vi "readdaq_tensions.vi"(10 "error in (no error)":errorcluster, 11 "Refnum in":refnum<k21>) -> (2 "viconsync":dbl, 3 "Tension Sensors Data":dbl[](array[numeric]), 5 "error out":errorcluster)   [LabVIEW 2017]
uses:
  <vilib>/DAQmx/read.llb/DAQmx Read (Analog 1D DBL NChan 1Samp).vi
  <vilib>/DAQmx/miscellaneous.llb/DAQmx Fill In Error Info.vi
  <vilib>/ptbypt/NI_PtbyPt.lvlib
panel:
  out "filtered":dbl[](array[numeric])
  out "Waveform Chart 2":dbl[](graph)
  in  "taresensors":bool
  out "raw data":dbl[](array[numeric]) format="%0.2f"
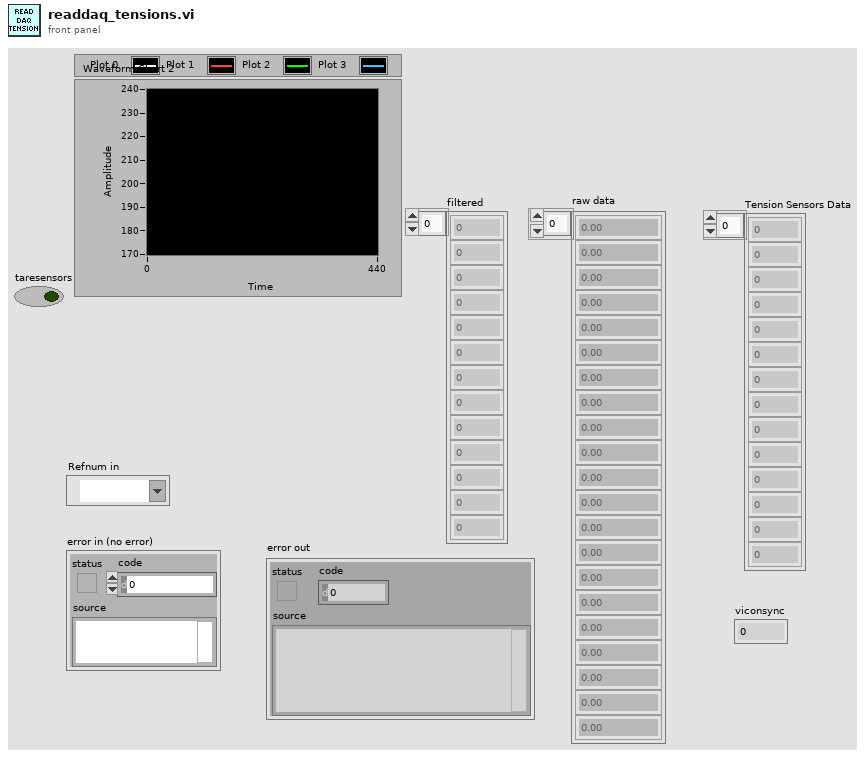
[diagram p1: front panel]
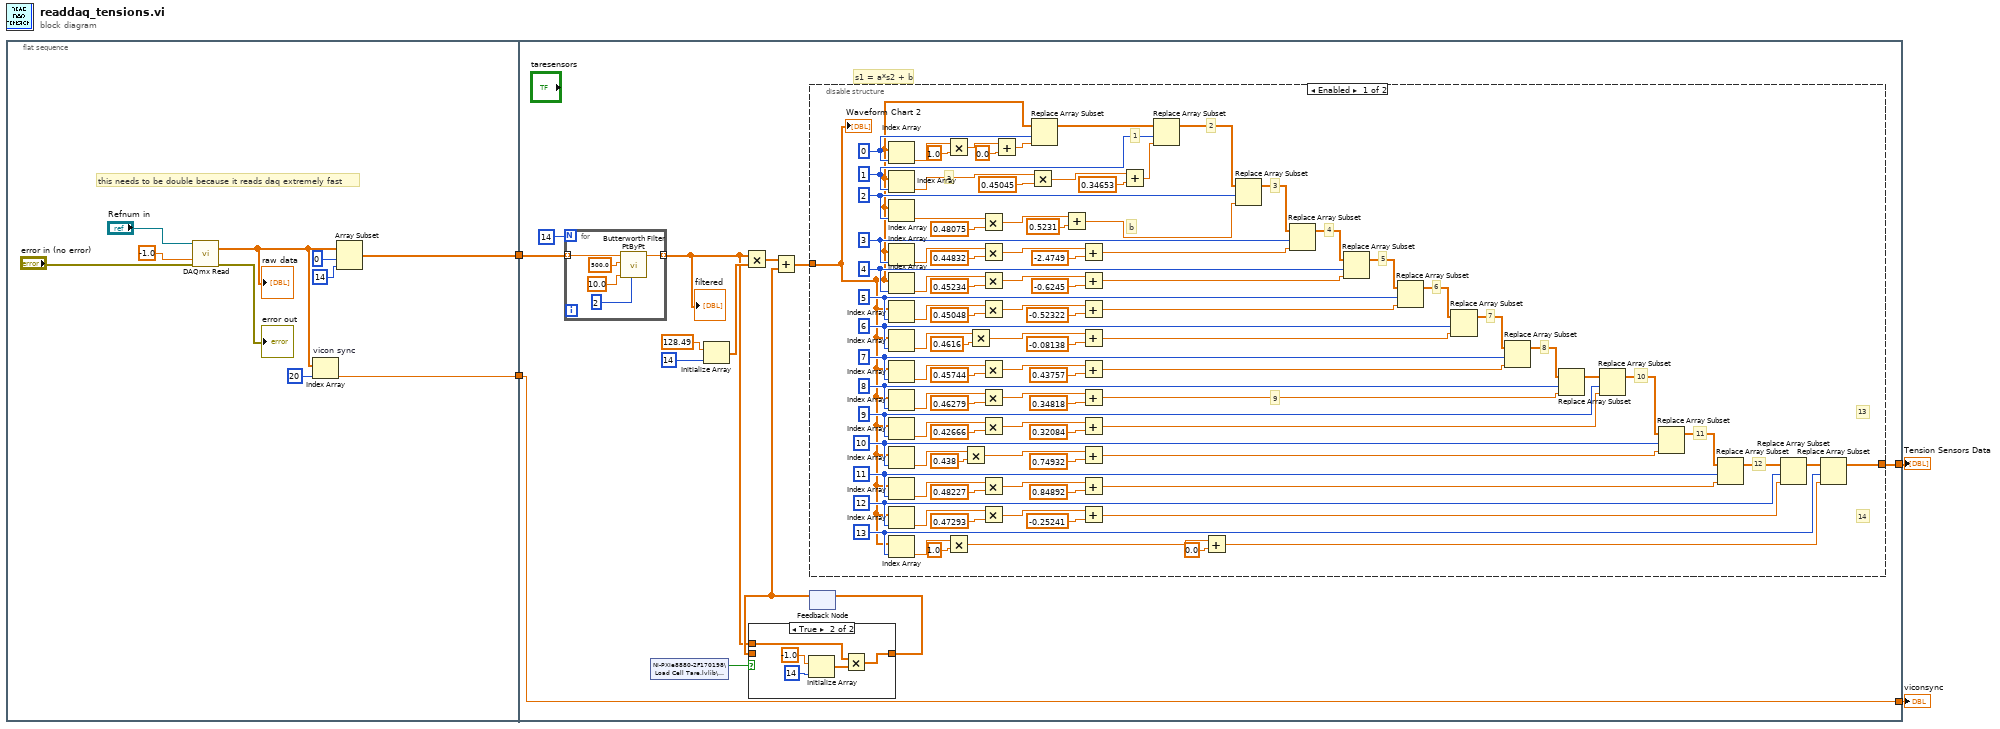
[diagram p0: block diagram]
diagram:
  n1 = flat-sequence {
    tunnel: [w8] -> w4
    tunnel: [w7] -> w3
    tunnel: w4 -> [w19]
    tunnel: w3 -> [w16]
    tunnel: [w20] -> w2
    tunnel: [w19] -> w1
    frame #0 {
      # "this needs to be double because it reads daq extremely fast"
      n2 = call-poly <vilib>:"DAQmx Read.vi"("task/channels in"="Refnum in", "timeout"=-1.0, "error in"="error in (no error)") -> ("data"=w10:dbl[], "error out"=→"error out":errorcluster)  [unwired: 10 in, 1 out]
      "raw data" <- w10
      n3 = Index Array "vicon sync"(array=w10, index=20) -> (element=w8:dbl)
      n4 = Array Subset(array=w10, index=0, length=14) -> (w7:dbl[])
    }
    frame #1 {
      # "s1 = a*s2 + b"
      n5 = for {
        N: 14 -> [_]
        tunnel: w16 -> [w32] mode=indexing
        tunnel: [w28] -> w15 mode=indexing
        n6 = call <vilib>:"Butterworth Filter PtByPt.vi"("order"=2, "low cutoff freq: fl"=10.0, "sampling freq: fs"=500.0, "x"=w32) -> ("Filtered x"=w28:dbl)  [unwired: 5 in, 1 out]
      }
      "filtered" <- w15
      n7 = shared-variable "NI-PXIe8880-2F170198\\Load Cell Tare.lvlib\\TareTrue"() -> (w18:bool)  [unwired: 1 in, 1 out]
      n8 = Initialize Array(128.49 ("element"), 14 ("dimension size")) -> (w25:dbl[])
      n9 = Multiply(x=w15, y=w25) -> (x*y=w24:dbl[])
      n10 = feedback #1() -> (w22:dbl[])  [unwired: 1 in]
      n11 = case shown="True" w18 {
        tunnel: w15 -> [_ w134]
        tunnel: [w132 w133] -> w23
        tunnel: w22 -> [w132 _]
        frame False {
        }
        frame True {
          n12 = Initialize Array(-1.0 ("element"), 14 ("dimension size")) -> (w137:dbl[])
          n13 = Multiply(x=w134, y=w137) -> (x*y=w133:dbl[])
        }
      }
      n14 = Add ("Add.vi")(x=w24, y=w22) -> (x+y=w21:dbl[])
      n15 = disable-structure shown="Enabled" {
        disable-tunnel: w21 -> [w44 _]
        disable-tunnel: [w43 _] -> w20
        frame Enabled {
          w47 = 13 ("index")
          w53 = 12 ("index")
          w59 = 11 ("index")
          w65 = 10 ("index")
          w71 = 9 ("index")
          w77 = 8 ("index")
          w83 = 7 ("index")
          w89 = 6 ("index")
          w95 = 5 ("index")
          w101 = 4 ("index")
          w116 = 3 ("index")
          w117 = 2 ("index")
          w118 = 1 ("index")
          w119 = 0 ("index")
          # "14"
          # "13"
          # "12"
          # "11"
          # "10"
          # "9"
          # "8"
          # "7"
          # "6"
          # "5"
          # "4"
          # "3"
          # "2"
          # "1"
          # "b"
          # "a"
          n16 = Index Array(array=w44, index=w119) -> (element=w108:dbl)
          n17 = Index Array(array=w44, index=w118) -> (element=w107:dbl)
          n18 = Index Array(array=w44, index=w117) -> (element=w106:dbl)
          n19 = Index Array(array=w44, index=w116) -> (element=w105:dbl)
          n20 = Index Array(array=w44, index=w101) -> (element=w99:dbl)
          n21 = Index Array(array=w44, index=w95) -> (element=w93:dbl)
          n22 = Index Array(array=w44, index=w89) -> (element=w87:dbl)
          n23 = Index Array(array=w44, index=w83) -> (element=w81:dbl)
          n24 = Index Array(array=w44, index=w77) -> (element=w75:dbl)
          n25 = Index Array(array=w44, index=w71) -> (element=w69:dbl)
          n26 = Index Array(array=w44, index=w65) -> (element=w63:dbl)
          n27 = Index Array(array=w44, index=w59) -> (element=w57:dbl)
          n28 = Index Array(array=w44, index=w53) -> (element=w51:dbl)
          n29 = Index Array(array=w44, index=w47) -> (element=w45:dbl)
          n30 = Multiply(x=w108, y=1.0) -> (x*y=w130:dbl)
          n31 = Multiply(x=w45, y=1.0) -> (x*y=w49:dbl)
          n32 = Multiply(x=w63, y=0.438) -> (x*y=w67:dbl)
          n33 = Multiply(x=w87, y=0.4616) -> (x*y=w91:dbl)
          n34 = Multiply(x=w106, y=0.48075) -> (x*y=w124:dbl)
          n35 = Multiply(x=w105, y=0.44832) -> (x*y=w121:dbl)
          n36 = Multiply(x=w99, y=0.45234) -> (x*y=w103:dbl)
          n37 = Multiply(x=w93, y=0.45048) -> (x*y=w97:dbl)
          n38 = Multiply(x=w81, y=0.45744) -> (x*y=w85:dbl)
          n39 = Multiply(x=w75, y=0.46279) -> (x*y=w79:dbl)
          n40 = Multiply(x=w69, y=0.42666) -> (x*y=w73:dbl)
          n41 = Multiply(x=w57, y=0.48227) -> (x*y=w61:dbl)
          n42 = Multiply(x=w51, y=0.47293) -> (x*y=w55:dbl)
          n43 = Add(x=w130, y=0.0) -> (x+y=w112:dbl)
          n44 = Multiply(x=w107, y=0.45045) -> (x*y=w127:dbl)
          n45 = Replace Array Subset(array=w44, new element=w112, index=w119) -> (w115:dbl[])
          n46 = Add(x=w124, y=0.5231) -> (x+y=w110:dbl)
          n47 = Add(x=w121, y=-2.4749) -> (x+y=w109:dbl)
          n48 = Add(x=w103, y=-0.6245) -> (x+y=w100:dbl)
          n49 = Add(x=w97, y=-0.52322) -> (x+y=w94:dbl)
          n50 = Add(x=w91, y=-0.08138) -> (x+y=w88:dbl)
          n51 = Add(x=w85, y=0.43757) -> (x+y=w82:dbl)
          n52 = Add(x=w79, y=0.34818) -> (x+y=w76:dbl)
          n53 = Add(x=w73, y=0.32084) -> (x+y=w70:dbl)
          n54 = Add(x=w67, y=0.74932) -> (x+y=w64:dbl)
          n55 = Add(x=w61, y=0.84892) -> (x+y=w58:dbl)
          n56 = Add(x=w55, y=-0.25241) -> (x+y=w52:dbl)
          n57 = Add(x=w127, y=0.34653) -> (x+y=w111:dbl)
          n58 = Replace Array Subset(array=w115, new element=w111, index=w118) -> (w114:dbl[])
          n59 = Add(x=w49, y=0.0) -> (x+y=w46:dbl)
          n60 = Replace Array Subset(array=w114, new element=w110, index=w117) -> (w113:dbl[])
          n61 = Replace Array Subset(array=w113, new element=w109, index=w116) -> (w42:dbl[])
          n62 = Replace Array Subset(array=w42, new element=w100, index=w101) -> (w41:dbl[])
          n63 = Replace Array Subset(array=w41, new element=w94, index=w95) -> (w40:dbl[])
          n64 = Replace Array Subset(array=w40, new element=w88, index=w89) -> (w39:dbl[])
          n65 = Replace Array Subset(array=w39, new element=w82, index=w83) -> (w38:dbl[])
          n66 = Replace Array Subset(array=w38, new element=w76, index=w77) -> (w37:dbl[])
          n67 = Replace Array Subset(array=w37, new element=w70, index=w71) -> (w36:dbl[])
          n68 = Replace Array Subset(array=w36, new element=w64, index=w65) -> (w35:dbl[])
          n69 = Replace Array Subset(array=w35, new element=w58, index=w59) -> (w34:dbl[])
          n70 = Replace Array Subset(array=w34, new element=w52, index=w53) -> (w33:dbl[])
          n71 = Replace Array Subset(array=w33, new element=w46, index=w47) -> (w43:dbl[])
          "Waveform Chart 2" <- w44
        }
        frame Disabled {
        }
      }
      n72 = feedback-in #1(w23) -> ()
    }
  }
  "Tension Sensors Data" <- w2
  "viconsync" <- w1
